vi "Get Setting - Show_Error_Window_Default.vi"(8 "Error In":errorcluster) -> (0 "Error Out":errorcluster, 3 "Show_Error_Window_Default":T1)   [LabVIEW 2023, in "Error Manager.lvlib" / "Settings.lvclass"]
uses:
  Settings.lvclass
  Settings.lvclass/Settings.ctl
  Settings (class variable).vi
  Show_Error_Window_Default (enum).ctl
panel:
  # "Input\nInputs to the VI"
  # "Development\nControls or indicators that are useful for development or testing, but which are not outputs of the VI."
  # "Output\nOutputs of the VI"
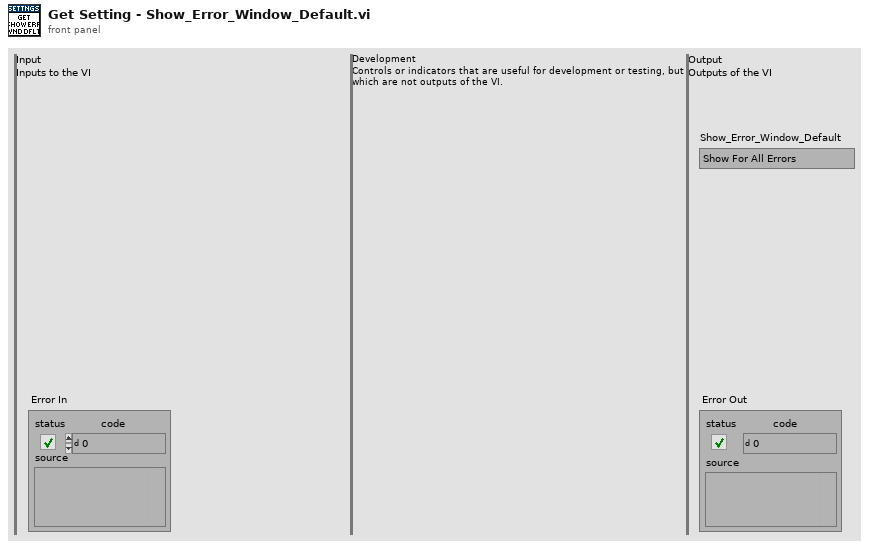
[diagram p1: front panel]
types:
  T1 = typedef "Error Manager.lvlib/Settings.lvclass/Show_Error_Window_Default (enum).ctl" = enum16{"Show For All Errors", "Show For New Errors", "Show For New Error Codes", "Do Not Show"}
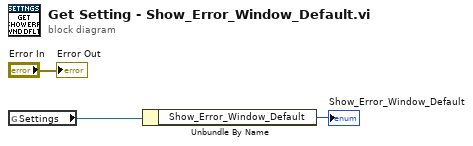
[diagram p0: block diagram]
diagram:
  n1 = global read "Settings (class variable).vi" "Settings"() -> (w1:refnum<class "Settings.lvclass">)
  n2 = Unbundle By Name(w1) -> ("Show_Error_Window_Default"=→"Show_Error_Window_Default":T1)
  "Error Out" <- "Error In"
